vi "Set Window Foreground.vi"(8 "error in (no error)":errorcluster, 11 "hWnd":i32) -> (0 "error out":errorcluster)   [LabVIEW 2020, in "PicoG-Processor.lvlib"]
uses:
  PicoG-Processor.lvlib
  <vilib>/Utility/error.llb/Error Cluster From Error Code.vi
  <vilib>/ErrorRing/Error Ring.xnode
  user32.dll
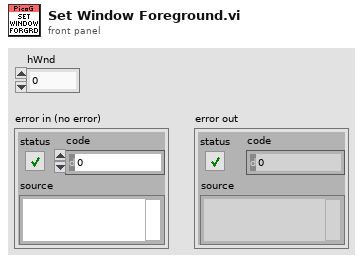
[diagram p1: front panel]
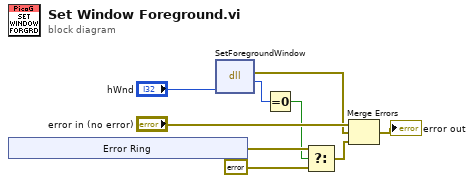
[diagram p0: block diagram]
diagram:
  n1 = xnode "Error Ring"() -> ("error out"=w5:errorcluster)
  n2 = dll-call lib="user32.dll" fn="SetForegroundWindow"("hWnd"="hWnd") -> (error out=w7:errorcluster, "return type"=w2:i8)  [unwired: 4 in, 1 out]
  n3 = Equal To 0?(x=w2) -> (x = 0?=w1:bool)
  n4 = Select(t=w5, s=w1, f=errorcluster {"status"=FALSE, "code"=0, "source"=""}) -> (s? t:f=w3:errorcluster)
  n5 = Merge Errors("error in (no error)", w7, w3) -> (→"error out":errorcluster)
